vi "Current_readings.vi"() -> ()   [LabVIEW 2017]
uses:
  <vilib>/Analysis/baseanly.llb/Mean (DBL).vi
  <instrlib>/Keithley 6517/Keithley 6517.lvlib
  <vilib>/Analysis/NI_AALBase.lvlib
panel:
  in  "V-source Amplitude (0.000000E+0)":dbl format="%.6e"
  out "error":i32
  out "mean":dbl format="%0.2f"
  out "Array":dbl[](array[numeric])
  in  "?":dbl
  in  "milliseconds to wait":u32
  out "error out 3":errorcluster
  in  "error in (no error) 3":errorcluster
  in  "VISA resource name 2":refnum<visa-resource-name>
  in  "error in (no error) 2":errorcluster
  out "VISA resource name out 2":refnum<visa-resource-name>
  out "error out 2":errorcluster
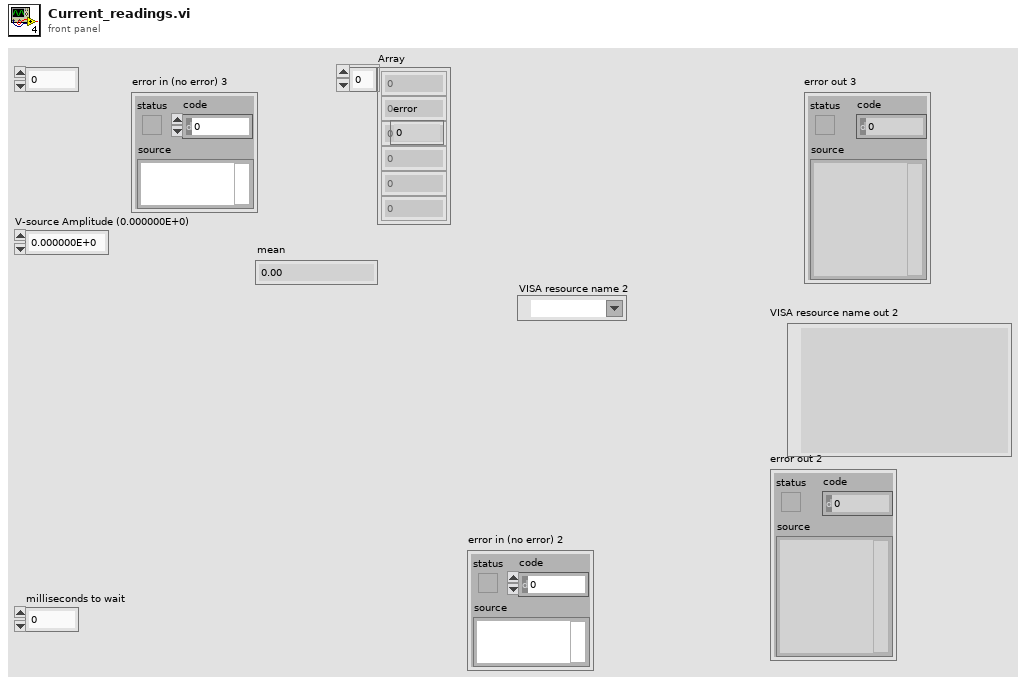
[diagram p1: front panel]
types:
  T1 = cluster{"Measurement":dbl, "Units":string, "Time Stamp and Date":string, "Reading #":dbl, "Channel #":dbl}
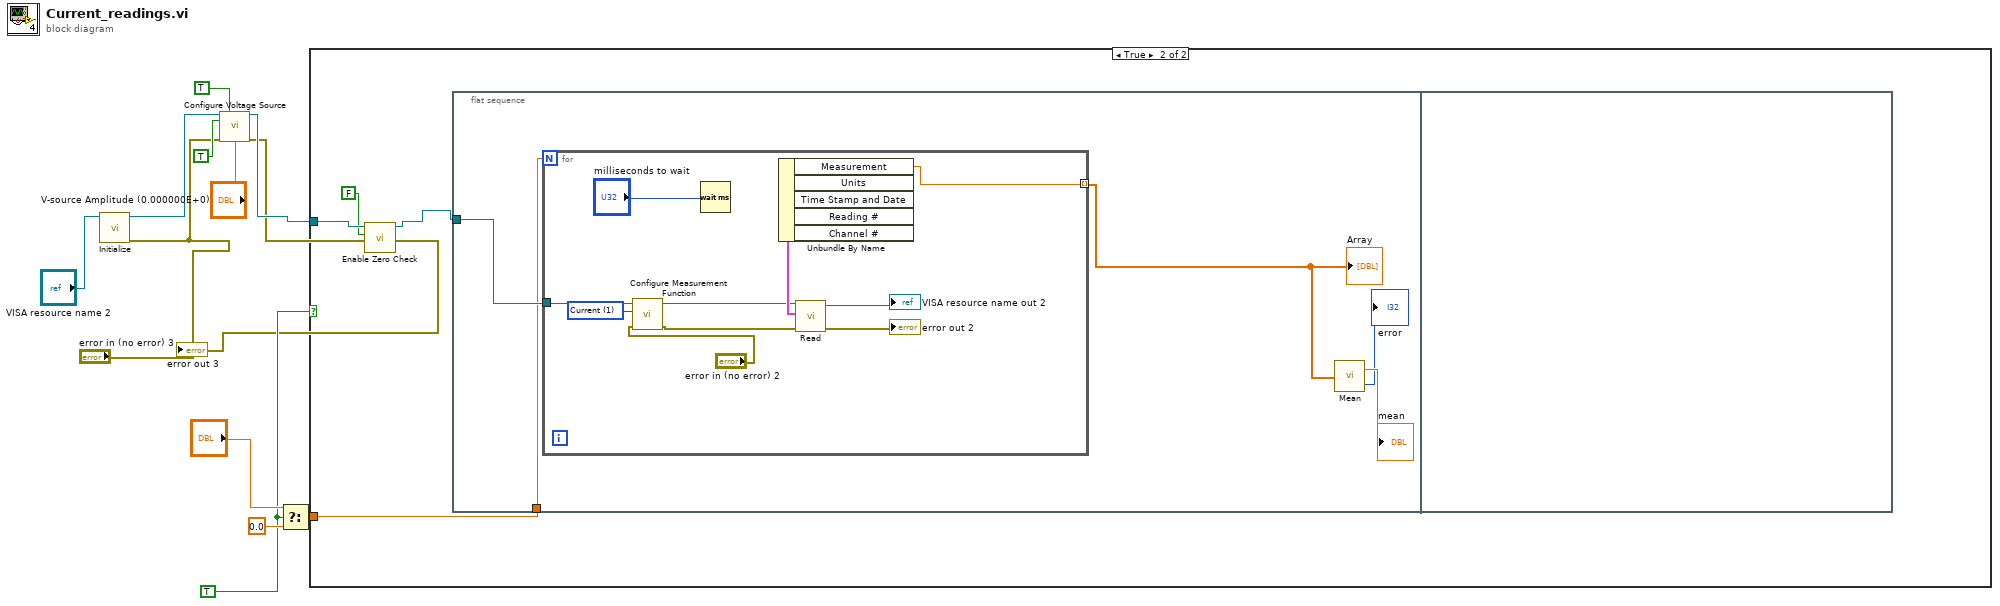
[diagram p0: block diagram]
diagram:
  w8 = TRUE
  n1 = call <instrlib>:"Initialize.vi"("error in (no error)"="error in (no error) 3", "VISA resource name"="VISA resource name 2") -> ("VISA resource name out"=w7:refnum<visa-resource-name>)  [unwired: 8 in, 1 out]
  n2 = call <instrlib>:"Configure Voltage Source.vi"("VISA resource name"=w7, "Enable LO Connection (F: Disable)"=TRUE, "Enable V-source (F: Disable)"=TRUE, "error in (no error)"="error in (no error) 3", "V-source Amplitude (0.000000E+0)"="V-source Amplitude (0.000000E+0)") -> ("VISA resource name out"=w6:refnum<visa-resource-name>, "error out"=→"error out 3":errorcluster)  [unwired: 9 in]
  n3 = Select(t="?", s=w8, f=0.0) -> (s? t:f=w10:dbl)
  n4 = case shown="True" w8 {
    tunnel: w6 -> [_ w15]
    tunnel: w10 -> [_ w16]
    frame False {
    }
    frame True {
      n5 = call <instrlib>:"Enable Zero Check.vi"("Enable Zero Check (T: Enable)"=FALSE, "VISA resource name"=w15) -> ("VISA resource name out"=w14:refnum<visa-resource-name>)  [unwired: 8 in, 1 out]
      n6 = flat-sequence {
        tunnel: w14 -> [w21]
        tunnel: w16 -> [w20]
        frame #0 {
          n7 = for {
            N: w20 -> [_]
            tunnel: w21 -> [w26]
            tunnel: [w27] -> w19 mode=indexing
            w24 = 1 items=["Voltage", "Current", "Resistance", "Charge"] ("Measurement Function (0: Voltage)")
            n8 = call <instrlib>:"Configure Measurement Function.vi"("error in (no error)"="error in (no error) 2", "Measurement Function (0: Voltage)"=w24, "VISA resource name"=w26) -> ("error out"=w22:errorcluster, "VISA resource name out"=w25:refnum<visa-resource-name>)  [unwired: 7 in]
            n9 = Wait (ms)(milliseconds to wait="milliseconds to wait") -> ()  [unwired: 1 out]
            n10 = call <instrlib>:"Read.vi"("error in (no error)"=w22, "VISA resource name"=w25) -> ("error out"=→"error out 2":errorcluster, "Measurement"=w28:T1, "VISA resource name out"=→"VISA resource name out 2":refnum<visa-resource-name>)  [unwired: 7 in]
            n11 = Unbundle By Name(w28) -> ("Measurement"=w27:dbl)  [unwired: 4 out]
          }
          "Array" <- w19
          n12 = call-poly <vilib>:"Mean.vi"("X"=w19) -> ("mean"=→"mean":dbl, "error"=→"error":i32)
        }
        frame #1 {
        }
      }
    }
  }
